vi "sample.vi"() -> ()   [LabVIEW 2013]
panel:
  out "time elapsed (ms)":u32
  in  "Boolean 2":bool
  in  "stop":bool
  out "Value":dbl
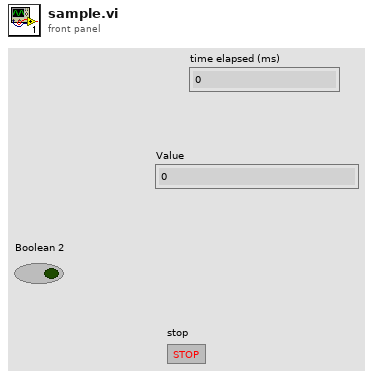
[diagram p1: front panel]
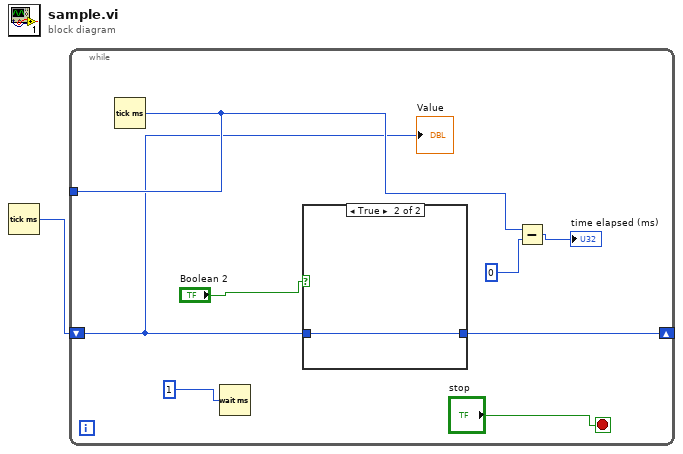
[diagram p0: block diagram]
diagram:
  n1 = Tick Count (ms)() -> (millisecond timer value=w1:u32)
  n2 = while {
    shift-right: [w7] -> _
    shift-left: w1 -> [w2]
    tunnel: [w4] -> _
    stop <- "stop" stop-if-true
    n3 = Tick Count (ms)() -> (millisecond timer value=w4:u32)
    n4 = Wait (ms)(milliseconds to wait=1) -> ()  [unwired: 1 out]
    n5 = case shown="True" "Boolean 2" {
      tunnel: w2 -> [w10 w11]
      tunnel: [w10 w11] -> w7
      frame False {
      }
      frame True {
      }
    }
    n6 = Subtract(x=w4, y=0) -> (x-y=→"time elapsed (ms)":u32)
    "Value" <- w2
  }
